vi "CodigoLabView 3.1.vi"() -> (11 "Releb 2":bool)   [LabVIEW 2025]
uses:
  <vilib>/Utility/NIReport.llb/Report Type.ctl
  <vilib>/Instr/_visa.llb/VISA Configure Serial Port (Instr).vi
  <vilib>/addons/_office/excel.llb/Excel Easy Table (str).vi
  <vilib>/Utility/NIReport.llb/NI_report.lvclass
  <vilib>/Utility/NIReport.llb/NI_ReportGenerationCore.lvlib
  <vilib>/addons/_office/NI_ReportGenerationToolkit.lvlib
  <vilib>/Utility/NIReport.llb/Excel/NI_Excel.lvclass
panel:
  out "TENSIÓN DE LÍNEA":dbl(knob) scale=100.0..300.0
  out "?":dbl(knob) scale=0.0..100.0
  out "?":dbl(knob) scale=0.0..100.0
  out "?":dbl(knob) scale=0.0..100.0
  out "?":dbl(knob) scale=0.0..100.0
  in  "?":bool
  out "Releb 4":bool
  out "Relea 4":bool
  out "Rele 4":bool
  out "Boolean 4":bool
  out "Estado 4":string
  in  "Relé N°4":bool
  out "POTENCIA":string
  out "Releb 3":bool
  out "Relea 3":bool
  out "Rele 3":bool
  out "Boolean 3":bool
  out "Estado 3":string
  out "POTENCIA":string
  in  "Relé N°3":bool
  out "Relea 2":bool
  out "Rele 2":bool
  out "TOMACORRIENTE 2":bool
  out "Estado 2":string
  out "POTENCIA":string
  in  "Relé N°2":bool
  out "Releb 1":bool
  out "Relea 1":bool
  out "Rele 1":bool
  out "TOMACORRIENTE 1":bool
  out "Estado 1":string
  out "POTENCIA":string
  in  "Relé N°1":bool
  in  "RUTA DE REGISTRO":path
  out "Tensión":string
  in  "PUERTO DE COMUNICACIÓN":refnum<visa-resource-name>
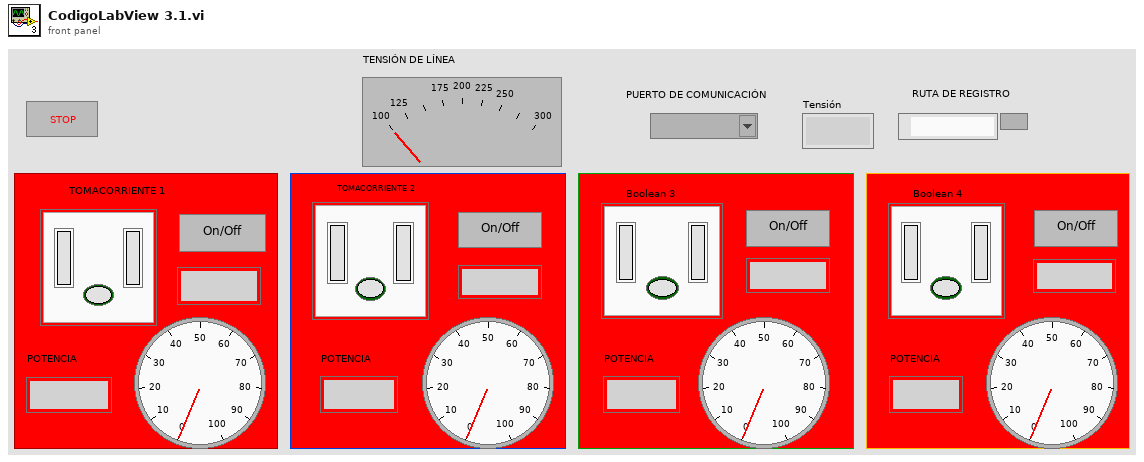
[diagram p1: front panel]
types:
  T1 = cluster{"W1":string, "W2":string, "W3":string, "W4":string, "V":string}
  T2 = typedef "NI_ReportGenerationCore.lvlib/Report Type.ctl" = enum16{"HTML", "Word", "Excel"}
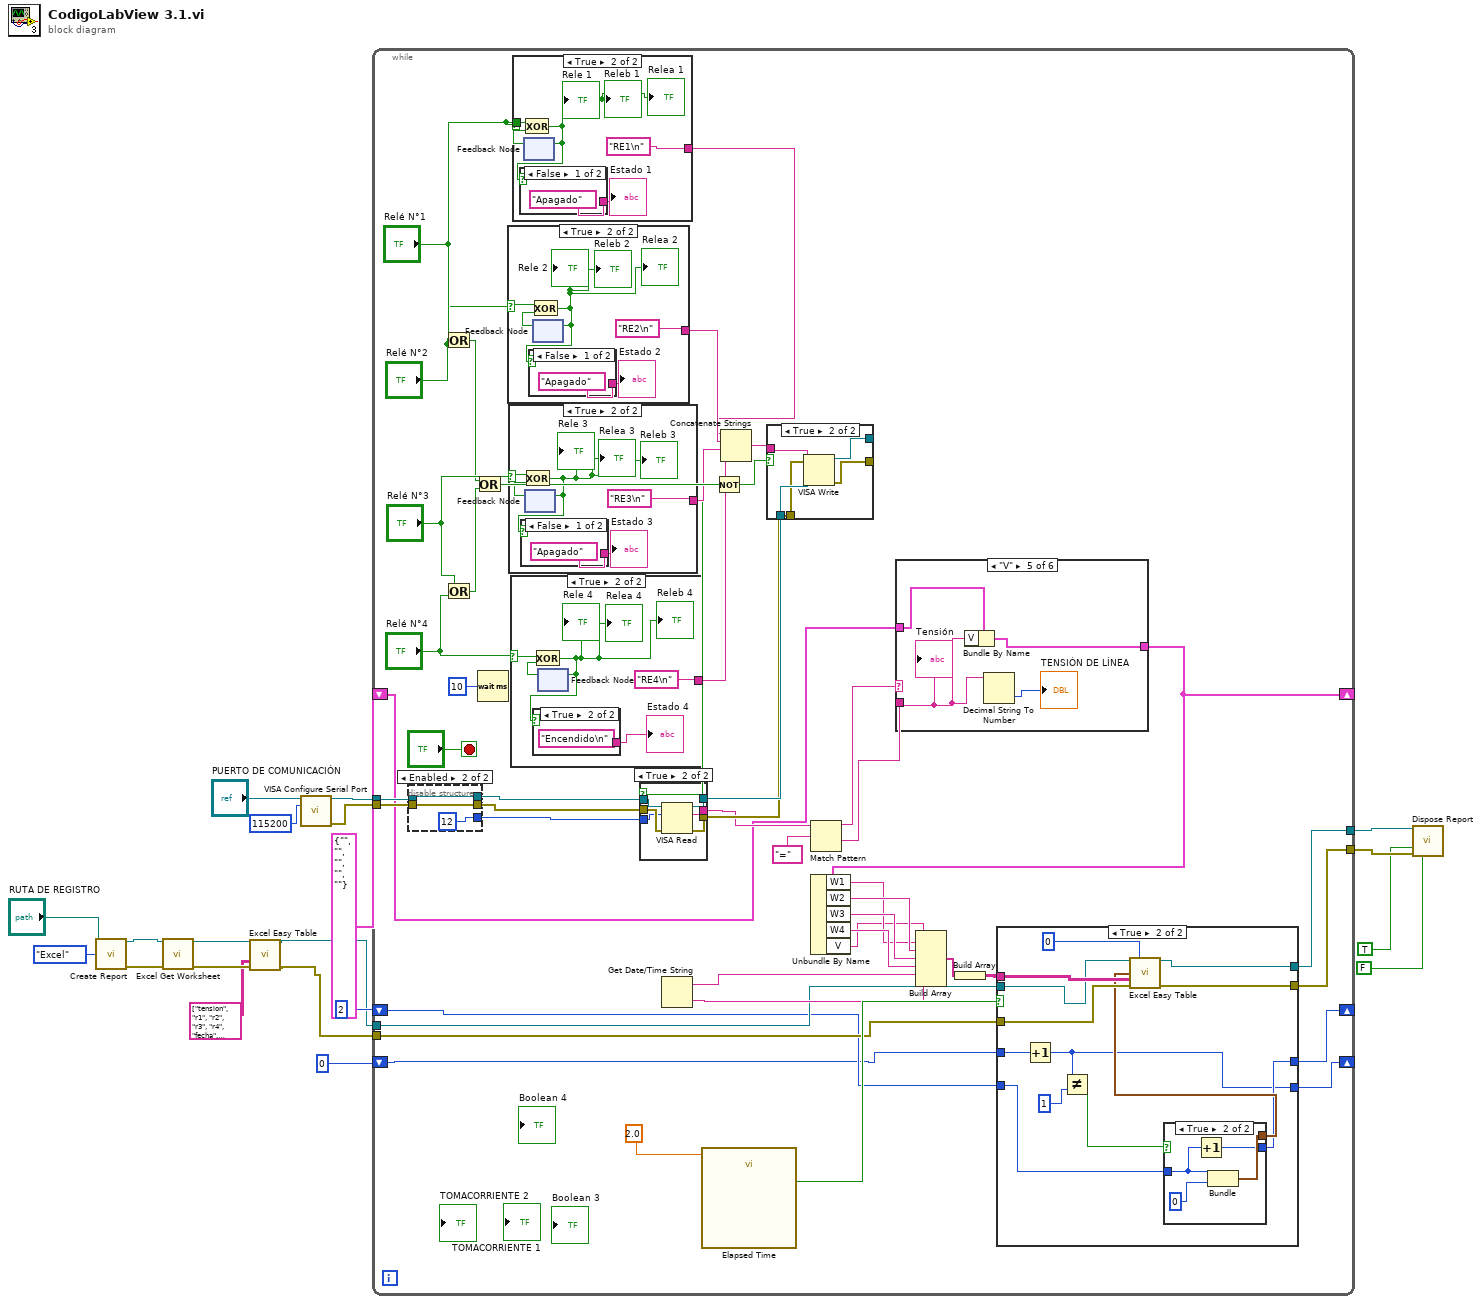
[diagram p0: block diagram]
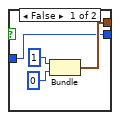
[diagram p3: hidden frame]
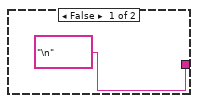
[diagram p4: hidden frame]
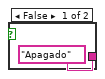
[diagram p5: hidden frame]
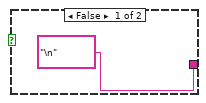
[diagram p6: hidden frame]
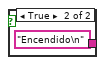
[diagram p7: hidden frame]
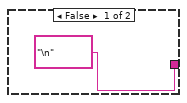
[diagram p8: hidden frame]
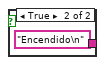
[diagram p9: hidden frame]
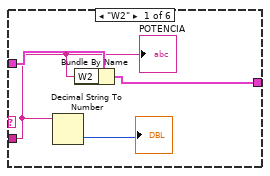
[diagram p10: hidden frame]
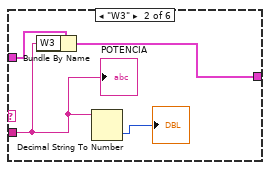
[diagram p11: hidden frame]
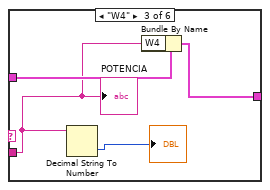
[diagram p12: hidden frame]
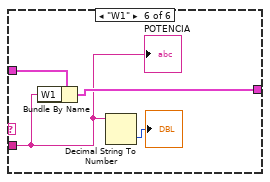
[diagram p14: hidden frame]
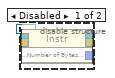
[diagram p15: hidden frame]
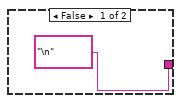
[diagram p18: hidden frame]
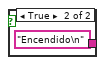
[diagram p19: hidden frame]
diagram:
  n1 = call <vilib>:"Create Report.vi"("report type"=Report_Type."Excel", "template (empty)"="RUTA DE REGISTRO") -> ("report out"=w10:refnum<class "NI_report.lvclass">, "error out"=w9:errorcluster)  [unwired: 12 in]
  n2 = call <vilib>:"Excel Get Worksheet.vi"("report in"=w10, "error in (no error)"=w9) -> ("report out"=w4:refnum<class "NI_report.lvclass">, "error out"=w3:errorcluster)  [unwired: 12 in]
  n3 = call-poly <vilib>:"Excel Easy Table.vi"("report in"=w4, "text data"=string[][] [["tension", "r1", "r2", "r3", "r4", "fecha", "hora"]], "error in (no error)"=w3) -> ("report out"=w5:refnum<class "NI_report.lvclass">, "error out"=w6:errorcluster)  [unwired: 8 in, 3 out]
  n4 = call-poly "VISA Configure Serial Port"("VISA resource name"="PUERTO DE COMUNICACIÓN", "baud rate (9600)"=u32 115200) -> ("VISA resource name out"=w20:refnum<visa-resource-name>, "error out"=w17:errorcluster)  [unwired: 12 in]
  n5 = while {
    tunnel: w20 -> [w67]
    tunnel: w17 -> [w66]
    tunnel: [w45] -> w14
    tunnel: [w44] -> w13
    tunnel: w5 -> [w38]
    tunnel: w6 -> [w37]
    shift-right: [w35] -> _
    shift-left: 2 -> [w36]
    shift-right: [w33] -> _
    shift-left: 0 -> [w34]
    shift-right: [w25] -> _
    shift-left: T1 {"W1"="", "W2"="", "W3"="", "W4"="", "V"=""} -> [w30]
    stop <- "?" stop-if-true
    n6 = disable-structure shown="Enabled" {
      disable-tunnel: w67 -> [w142 w145]
      disable-tunnel: w66 -> [w141 w144]
      disable-tunnel: [w140 w145] -> w63
      disable-tunnel: [w139 u32 12 ("Bytes at Port")] -> w62
      disable-tunnel: [w138 w144] -> w61
      frame Disabled {
        n7 = property class="Instr"(reference=w142, error in=w141) -> (reference out=w140:refnum<visa-resource-name>, error out=w138:errorcluster, "Serial Settings:Number of Bytes at Serial Port"=w139:u32)
      }
      frame Enabled {
      }
    }
    n8 = Or(x="Relé N°1", y="Relé N°2") -> (x .or. y?=w52:bool)
    n9 = Or(x="Relé N°3", y="Relé N°4") -> (x .or. y?=w51:bool)
    n10 = Or(x=w52, y=w51) -> (x .or. y?=w56:bool)
    n11 = Wait (ms)(milliseconds to wait=u32 10) -> ()  [unwired: 1 out]
    n12 = case shown="True" "Relé N°2" {
      selector: "Relé N°2" -> [_ w111]
      tunnel: ["\n" "RE2\n"] -> w48
      frame False {
      }
      frame True {
        n13 = feedback #1() -> (w113:bool)  [unwired: 1 in]
        n14 = Exclusive Or(1:w113, 2:w111) -> (0:w110:bool)
        "Rele 2" <- w110
        "Releb 2" <- w110
        "Relea 2" <- w110
        n15 = case shown="False" w110 {
          tunnel: ["Apagado" "Encendido\n"] -> w112
          frame False {
          }
          frame True {
          }
        }
        "Estado 2" <- w112
        n16 = feedback-in #1(w110) -> ()
      }
    }
    n17 = case shown="True" "Relé N°3" {
      selector: "Relé N°3" -> [_ w103]
      tunnel: ["\n" "RE3\n"] -> w50
      frame False {
      }
      frame True {
        n18 = feedback #2() -> (w105:bool)  [unwired: 1 in]
        n19 = Exclusive Or(1:w105, 2:w103) -> (0:w102:bool)
        "Releb 3" <- w102
        "Relea 3" <- w102
        "Rele 3" <- w102
        n20 = case shown="False" w102 {
          tunnel: ["Apagado" "Encendido\n"] -> w104
          frame False {
          }
          frame True {
          }
        }
        "Estado 3" <- w104
        n21 = feedback-in #2(w102) -> ()
      }
    }
    n22 = case shown="True" "Relé N°4" {
      selector: "Relé N°4" -> [_ w95]
      tunnel: ["\n" "RE4\n"] -> w49
      frame False {
      }
      frame True {
        n23 = feedback #3() -> (w97:bool)  [unwired: 1 in]
        n24 = Exclusive Or(1:w97, 2:w95) -> (0:w94:bool)
        "Rele 4" <- w94
        "Releb 4" <- w94
        "Relea 4" <- w94
        n25 = case shown="True" w94 {
          tunnel: ["Apagado" "Encendido\n"] -> w96
          frame False {
          }
          frame True {
          }
        }
        "Estado 4" <- w96
        n26 = feedback-in #3(w94) -> ()
      }
    }
    n27 = case shown="True" "Relé N°1" {
      tunnel: ["\n" "RE1\n"] -> w22
      tunnel: "Relé N°1" -> [_ w165]
      frame False {
      }
      frame True {
        n28 = feedback #4() -> (w164:bool)  [unwired: 1 in]
        n29 = Exclusive Or(1:w164, 2:w165) -> (0:w162:bool)
        "Rele 1" <- w162
        "Relea 1" <- w162
        "Releb 1" <- w162
        n30 = case shown="False" w162 {
          tunnel: ["Apagado" "Encendido\n"] -> w163
          frame False {
          }
          frame True {
          }
        }
        "Estado 1" <- w163
        n31 = feedback-in #4(w162) -> ()
      }
    }
    n32 = Get Date/Time String() -> (date string=w40:string, time string=w39:string)  [unwired: 3 in]
    n33 = call "Elapsed Time"("Time Target (s)"=2.0) -> ("Time has Elapsed"=w41:bool)  [unwired: 11 in, 7 out]
    n34 = Not(x=w56) -> (.not. x?=w43:bool)
    n35 = case shown="True" w43 {
      tunnel: [w147 w153] -> w65
      tunnel: [w146 w152] -> w64
      tunnel: w61 -> [w146 w151]
      tunnel: w63 -> [w147 w150]
      tunnel: w62 -> [_ w149]
      tunnel: [_ w148] -> w32
      frame False {
      }
      frame True {
        n36 = VISA Read(VISA resource name=w150, byte count=w149, error in (no error)=w151) -> (VISA resource name out=w153:refnum<visa-resource-name>, read buffer=w148:string, error out=w152:errorcluster)  [unwired: 1 out]
      }
    }
    n37 = Concatenate Strings(w22, w48, w50, w49) -> (w23:string)
    n38 = case shown="True" w56 {
      tunnel: [w155 w160] -> _
      tunnel: [w154 w159] -> _
      tunnel: w65 -> [w155 w158]
      tunnel: w64 -> [w154 w157]
      tunnel: w23 -> [_ w156]
      frame False {
      }
      frame True {
        n39 = VISA Write(VISA resource name=w158, write buffer=w156, error in (no error)=w157) -> (VISA resource name out=w160:refnum<visa-resource-name>, error out=w159:errorcluster)  [unwired: 1 out]
      }
    }
    n40 = Match Pattern(string=w32, regular expression="=") -> (before substring=w58:string, after substring=w31:string)  [unwired: 1 in, 2 out]
    n41 = case shown="\"V\"" w58 {
      tunnel: w31 -> [w118 w122 w125 _ w130 w134]
      tunnel: w30 -> [w120 w124 w127 w129 w133 w137]
      tunnel: [w119 w123 w128 w129 w132 w136] -> w25
      frame "W2" {
        n42 = Decimal String To Number(string=w118) -> (number=→"?":i32)  [unwired: 2 in, 1 out]
        n43 = Bundle By Name(cluster=w120, "W2"=w118) -> (w119:T1)
        "POTENCIA" <- w118
      }
      frame "W3" {
        n44 = Bundle By Name(cluster=w124, "W3"=w122) -> (w123:T1)
        n45 = Decimal String To Number(string=w122) -> (number=→"?":i32)  [unwired: 2 in, 1 out]
        "POTENCIA" <- w122
      }
      frame "W4" {
        n46 = Decimal String To Number(string=w125) -> (number=→"?":i32)  [unwired: 2 in, 1 out]
        n47 = Bundle By Name(cluster=w127, "W4"=w125) -> (w128:T1)
        "POTENCIA" <- w125
      }
      frame "False", Default {
      }
      frame "V" {
        n48 = Bundle By Name(cluster=w133, "V"=w130) -> (w132:T1)
        n49 = Decimal String To Number(string=w130) -> (number=→"TENSIÓN DE LÍNEA":i32)  [unwired: 2 in, 1 out]
        "Tensión" <- w130
      }
      frame "W1" {
        n50 = Bundle By Name(cluster=w137, "W1"=w134) -> (w136:T1)
        n51 = Decimal String To Number(string=w134) -> (number=→"?":i32)  [unwired: 2 in, 1 out]
        "POTENCIA" <- w134
      }
    }
    n52 = Unbundle By Name(w25) -> ("W1"=w26:string, "W2"=w27:string, "W3"=w28:string, "W4"=w29:string, "V"=w24:string)
    n53 = Build Array(w24, w26, w27, w28, w29, w40, w39) -> (w47:string[])
    n54 = Build Array(w47) -> (w46:string[][])
    n55 = case shown="True" w41 {
      tunnel: w46 -> [_ w84]
      tunnel: w37 -> [w71 w83]
      tunnel: [w70 w82] -> w45
      tunnel: [w71 w81] -> w44
      tunnel: w38 -> [w70 w80]
      tunnel: w36 -> [w69 w77]
      tunnel: [w69 w76] -> w35
      tunnel: w34 -> [w68 w75]
      tunnel: [w68 w72] -> w33
      frame False {
      }
      frame True {
        n56 = Increment(x=w75) -> (x+1=w72:i32)
        n57 = Not Equal?(x=w72, y=1) -> (x != y?=w73:bool)
        n58 = case shown="True" w73 {
          tunnel: [w86 w92] -> w79
          tunnel: w77 -> [w85 w90]
          tunnel: [w85 w89] -> w76
          frame False {
            n59 = Bundle(1, 0) -> (w86:cluster{i32, i32})  [unwired: 1 in]
          }
          frame True {
            n60 = Increment(x=w90) -> (x+1=w89:i32)
            n61 = Bundle(w90, 0) -> (w92:cluster{i32, i32})  [unwired: 1 in]
          }
        }
        n62 = call-poly <vilib>:"Excel Easy Table.vi"("report in"=w80, "iteration"=0, "start (0, 0)"=w79, "text data"=w84, "error in (no error)"=w83) -> ("report out"=w82:refnum<class "NI_report.lvclass">, "error out"=w81:errorcluster)  [unwired: 6 in, 3 out]
      }
    }
  }
  n63 = call-dynamic "Dispose Report.vi"("report in"=w14, "save changes? (F)"=TRUE, "error in (no error)"=w13, "close report? (T)"=FALSE) -> ()  [unwired: 11 in, 1 out]
